vi "Override Direction.vi"(8 "error in (no error)":errorcluster, 10 "Direction":T1, 11 "Mock Transfer Group in":refnum<class "Mock Transfer Group.lvclass">) -> (0 "error out":errorcluster, 3 "Mock Transfer Group out":refnum<class "Mock Transfer Group.lvclass">)   [LabVIEW 2017, in "Mock Transfer Group.lvclass"]
uses:
  Mock Transfer Group.lvclass
  C:/Git/DSF/Data Sharing Framework Core/Classes/Transfer Group/Transfer Group.lvclass
  Typedefs/DSF Direction.ctl
  Classes/Transfer Group/Transfer Group.lvclass/Transfer Group.ctl
  Classes/Transfer Group/Transfer Group.lvclass
  DSF Core.lvlib
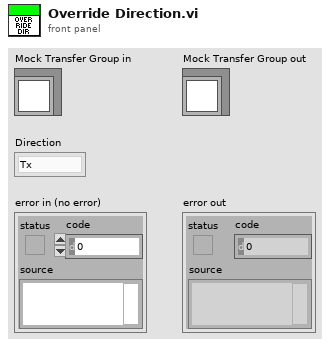
[diagram p1: front panel]
types:
  T1 = typedef "DSF Core.lvlib/DSF Direction.ctl" = enum8{"Tx", "Rx"}
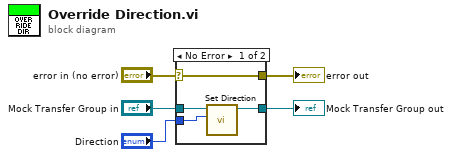
[diagram p0: block diagram]
diagram:
  n1 = case shown="No Error" "error in (no error)" {
    selector: "error in (no error)" -> [w9 w11]
    tunnel: [w9 w11] -> w4
    tunnel: [w7 w10] -> w2
    tunnel: "Mock Transfer Group in" -> [w8 w10]
    tunnel: "Direction" -> [w6 _]
    frame No Error {
      n2 = call "Set Direction.vi"("Direction"=w6, "Transfer Group in"=w8) -> ("Transfer Group out"=w7:refnum<class "Mock Transfer Group.lvclass">)  [unwired: 9 in]
    }
    frame Error {
    }
  }
  "error out" <- w4
  "Mock Transfer Group out" <- w2
